vi "Read IFD Entry from file.vi"(7 "Litt/BigEnd":bool, 8 "error in":errorcluster, 10 "Tag location in":i64, 11 "File":refnum<file>) -> (0 "error out":errorcluster, 2 "Next Tag location Out\n(IN + 12)":i64, 3 "File":refnum<file>, 4 "Tag":T1)   [LabVIEW 2013, in "Tiff reader.lvlib"]
doc: "Reads the next tag entry in the Image File Directory in a tiff file byte stream, returning the tag, its format and location in the byte stream."
uses:
  Tiff reader.lvlib
  IFD Entry.ctl
  FieldTypes.ctl
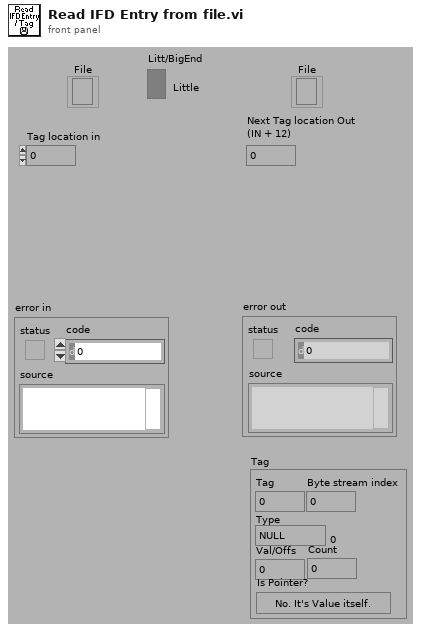
[diagram p1: front panel]
types:
  T1 = typedef "Tiff reader.lvlib/IFD Entry.ctl" = cluster{"Tag":u16, "Type":T2, "Count":u32, "Val/Offs":u32, "Is Pointer?":bool, "Byte stream index":i32}
  T2 = typedef "Tiff reader.lvlib/FieldTypes.ctl" = enum16{"NULL", "U8", "ASCII7", "U16", "U32", "RATIONAL", "SByte(I8)", "Undef(8Bit)", "I16", "I32", "SRat(4B:4B)", "SGL(4Byte)", "DBL(8Byte)"}
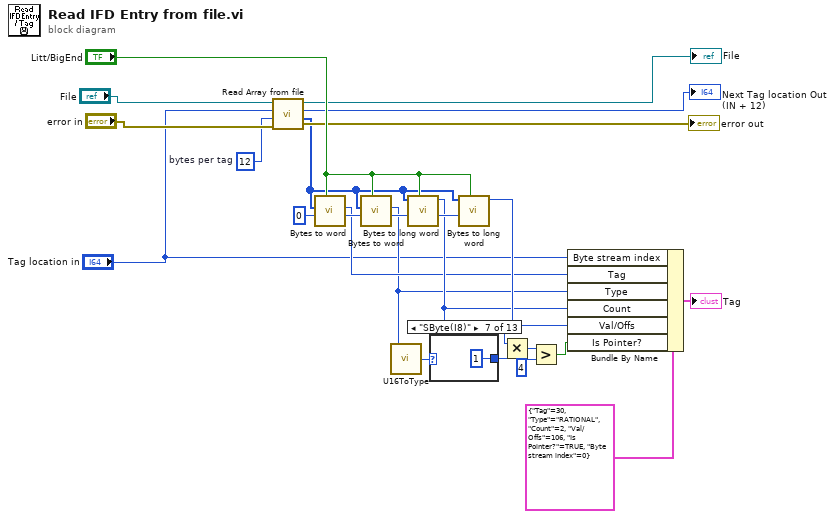
[diagram p0: block diagram]
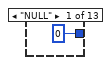
[diagram p2: hidden frame]
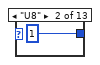
[diagram p3: hidden frame]
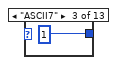
[diagram p4: hidden frame]
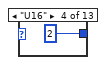
[diagram p5: hidden frame]
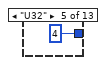
[diagram p6: hidden frame]
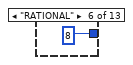
[diagram p7: hidden frame]
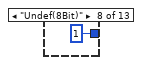
[diagram p8: hidden frame]
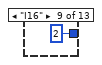
[diagram p9: hidden frame]
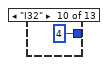
[diagram p10: hidden frame]
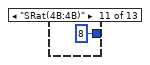
[diagram p11: hidden frame]
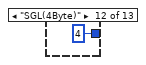
[diagram p12: hidden frame]
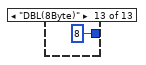
[diagram p13: hidden frame]
diagram:
  w3 = 12  # bytes per tag
  n1 = call "Read Array from file.vi"("error in"="error in", "bytes to read"=w3, "File location in"="Tag location in", "File"="File") -> ("error out"=→"error out":errorcluster, "Array of U8s"=w1:u8[], "File location after array read"=→"Next Tag location Out\n(IN + 12)":i64, "File out"=→"File":refnum<file>)
  n2 = call "Bytes to word.vi"("Litt/BigEnd"="Litt/BigEnd", "Index"=0, "Image Data in"=w1) -> ("Index+2"=w22:i32, "Word"=w12:u16)  [unwired: 1 in, 4 out]
  n3 = call "Bytes to word.vi"("Litt/BigEnd"="Litt/BigEnd", "Index"=w22, "Image Data in"=w1) -> ("Index+2"=w21:i32, "Word"=w11:u16)  [unwired: 1 in, 4 out]
  n4 = call "U16ToType.vi"("U16 In"=w11) -> ("Type out"=w18:T2)  [unwired: 4 out]
  n5 = call "Bytes to long word.vi"("Litt/BigEnd"="Litt/BigEnd", "Index"=w21, "Image Data in"=w1) -> ("Index+4"=w20:i32, "U32"=w16:u32)  [unwired: 5 out]
  n6 = case shown="\"SByte(I8)\"" w18 {
    tunnel: [i64 0 i64 1 i64 1 i64 2 i64 4 i64 8 i64 1 i64 1 i64 2 i64 4 i64 8 i64 4 i64 8] -> w17
    frame "NULL" {
    }
    frame "U8" {
    }
    frame "ASCII7" {
    }
    frame "U16" {
    }
    frame "U32" {
    }
    frame "RATIONAL" {
    }
    frame "SByte(I8)" {
    }
    frame "Undef(8Bit)" {
    }
    frame "I16" {
    }
    frame "I32" {
    }
    frame "SRat(4B:4B)" {
    }
    frame "SGL(4Byte)" {
    }
    frame "DBL(8Byte)" {
    }
  }
  n7 = call "Bytes to long word.vi"("Litt/BigEnd"="Litt/BigEnd", "Index"=w20, "Image Data in"=w1) -> ("U32"=w19:u32)  [unwired: 6 out]
  n8 = Multiply(x=w16, y=w17) -> (x*y=w15:i64)
  n9 = Greater?(x=w15, y=i64 4) -> (0:w13:bool)
  n10 = Bundle By Name(cluster=T1 {"Tag"=30, "Type"=enum."RATIONAL", "Count"=2, "Val/Offs"=106, "Is Pointer?"=TRUE, "Byte stream index"=0} ("Cluster"), "Byte stream index"="Tag location in", "Tag"=w12, "Type"=w11, "Count"=w16, "Val/Offs"=w19, "Is Pointer?"=w13) -> (→"Tag":T1)
